vi "VarexLib_Prompt.vi"(8 "error in (no error)":errorcluster, 10 "AD Group In":string) -> (0 "error out":errorcluster, 2 "OK?":bool, 3 "UserID Out":string)   [LabVIEW 2024]
uses:
  C:/Users/bjames/Documents/GitHub/DataLogger/SubVIs/VarexLib.dll
  DataLogger/SubVIs/VarexLib.dll
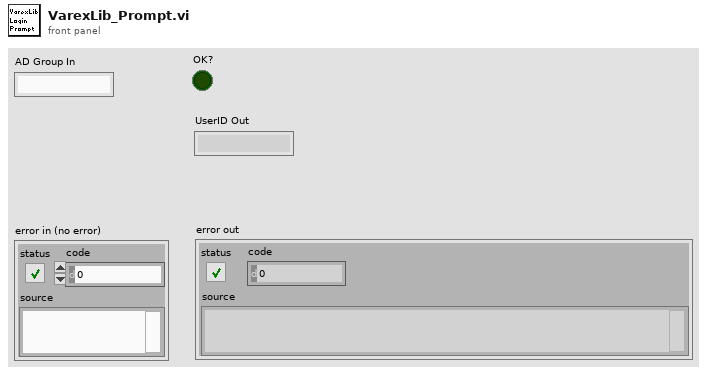
[diagram p1: front panel]
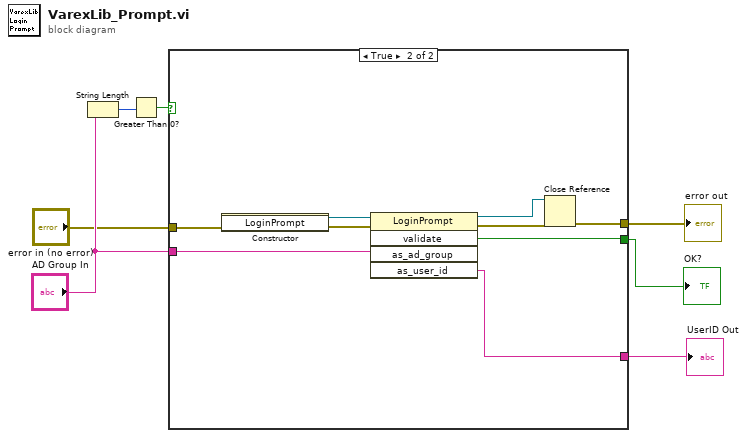
[diagram p0: block diagram]
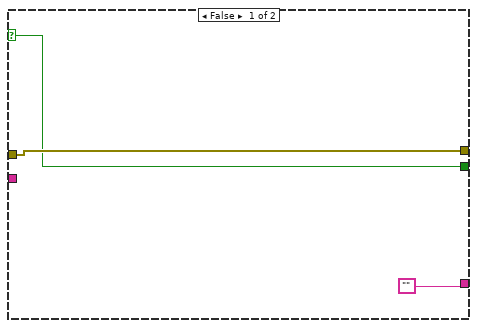
[diagram p2: hidden frame]
diagram:
  n1 = String Length(string="AD Group In") -> (length=w7:i32)
  n2 = Greater Than 0?(x=w7) -> (x > 0?=w6:bool)
  n3 = case shown="True" w6 {
    selector: w6 -> [w9 _]
    tunnel: "AD Group In" -> [_ w15]
    tunnel: "error in (no error)" -> [w10 w19]
    tunnel: [w10 w18] -> w3
    tunnel: [w9 w14] -> w2
    tunnel: ["" w13] -> w1
    frame False {
    }
    frame True {
      n4 = constructor class="LoginPrompt"(error in=w19) -> (reference out=w17:refnum<k24>, error out=w16:errorcluster)  [unwired: 2 in, 1 out]
      n5 = invoke class="LoginPrompt" method="validate"(reference=w17, error in=w16, "as_ad_group"=w15) -> (reference out=w11:refnum<k24>, error out=w12:errorcluster, "validate"=w14:bool, "as_user_id"=w13:string)  [unwired: 2 in, 1 out]
      n6 = Close Reference(reference=w11, error in (no error)=w12) -> (error out=w18:errorcluster)
    }
  }
  "error out" <- w3
  "OK?" <- w2
  "UserID Out" <- w1
